vi "Index_Array_1D.vi"(9 "Index Array 1D":i8[](array[numeric])=[1, 3, 4, -2, 0, 10], 10 "Index":i32) -> (2 "Value":i8)   [LabVIEW 2018]
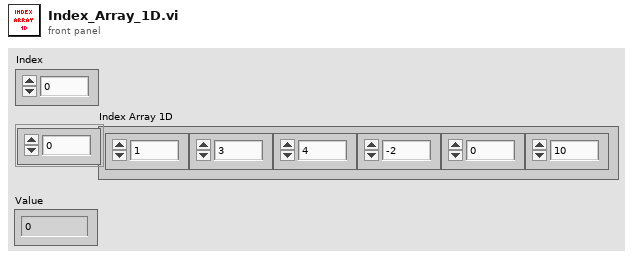
[diagram p1: front panel]
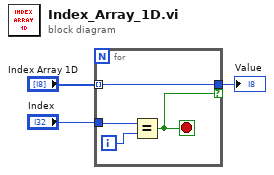
[diagram p0: block diagram]
diagram:
  n1 = for {
    tunnel: "Index Array 1D" -> [w5] mode=indexing
    tunnel: "Index" -> [w6]
    tunnel: [w5] -> w1 if=w4
    i -> [w7]
    stop <- w4 stop-if-true
    n2 = Equal?(x=w6, y=w7) -> (x = y?=w4:bool)
  }
  "Value" <- w1
